vi "tearDown.vi"(8 "error in (no error)":errorcluster, 11 "reference in":refnum<class "DSF CD GE Reflective Memory System Tests.lvclass">) -> (0 "error out":errorcluster, 3 "reference out":refnum<class "DSF CD GE Reflective Memory System Tests.lvclass">)   [LabVIEW 2017, in "DSF CD GE Reflective Memory System Tests.lvclass"]
doc: "tearDown runs after the test method has completed. Use this method to clean up any operations or references that were opened by setUp or the test method. Unit tests should be independent of other unit tests so this VI should ensure that the next test can run in a 'clean' test environment."
uses:
  DSF CD GE Reflective Memory System Tests.lvclass
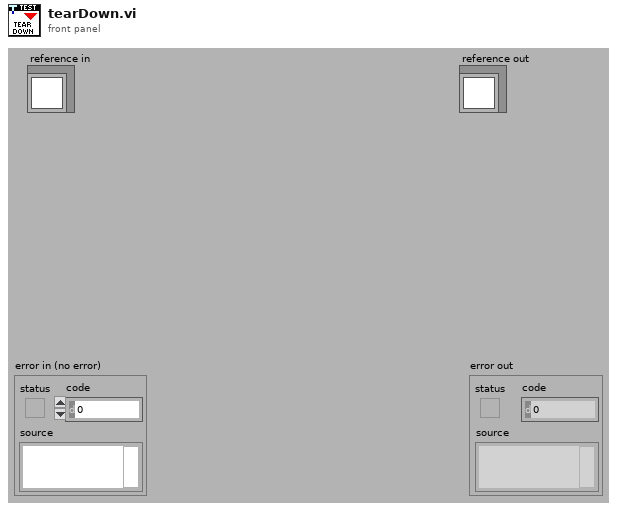
[diagram p1: front panel]
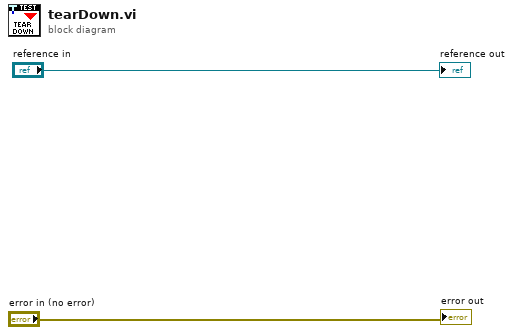
[diagram p0: block diagram]
diagram:
  "error out" <- "error in (no error)"
  "reference out" <- "reference in"
